vi "ACK_TAREA.vi"(8 "error in (no error)":errorcluster, 10 "Enum":T1, 11 "VISA resource name":refnum<visa-resource-name>) -> (0 "error out":errorcluster, 3 "read buffer":string)   [LabVIEW 2019]
uses:
  Type_defs/COMANDOS_TAREA.ctl
  <vilib>/Utility/error.llb/Error Cluster From Error Code.vi
  <vilib>/ErrorRing/Error Ring.xnode
panel:
  out "VISA resource name out":refnum<visa-resource-name>
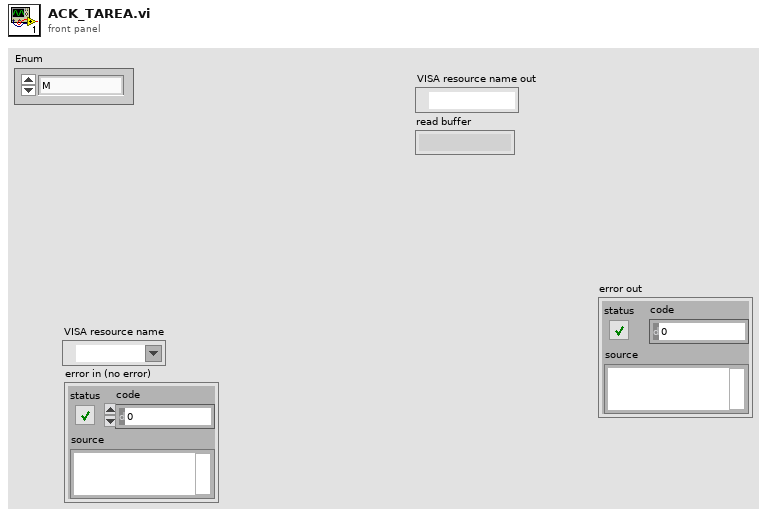
[diagram p1: front panel]
types:
  T1 = typedef "COMANDOS_TAREA.ctl" = enum16{"M", "T", "Q", "U", "S"}
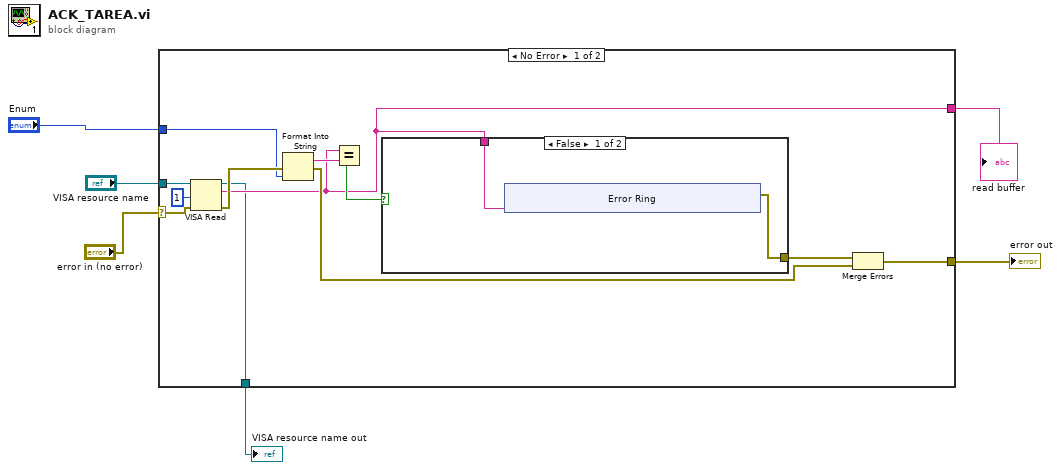
[diagram p0: block diagram]
diagram:
  n1 = case shown="No Error" "error in (no error)" {
    selector: "error in (no error)" -> [w9 w29]
    tunnel: "VISA resource name" -> [w18 w28]
    tunnel: [w12 _] -> w5
    tunnel: [w10 w29] -> w4
    tunnel: [w8 w28] -> w2
    tunnel: "Enum" -> [w7 _]
    frame No Error {
      n2 = VISA Read(VISA resource name=w18, byte count=u32 1, error in (no error)=w9) -> (VISA resource name out=w8:refnum<visa-resource-name>, read buffer=w12:string, error out=w14:errorcluster)  [unwired: 1 out]
      n3 = Format Into String(error in=w14, w7) -> (resulting string=w16:string, error out=w13:errorcluster)  [unwired: 2 in]
      n4 = Equal?(x=w12, y=w16) -> (x = y?=w15:bool)
      n5 = case shown="False" w15 {
        tunnel: w12 -> [w20 _]
        tunnel: [w19 _] -> w11
        frame False {
          n6 = xnode ("Error Ring")("parameter 0"=w20) -> ("error out"=w19:errorcluster)
        }
        frame True {
        }
      }
      n7 = Merge Errors(w11, w13) -> (w10:errorcluster)
    }
    frame Error {
    }
  }
  "error out" <- w4
  "VISA resource name out" <- w2
  "read buffer" <- w5
